vi "All on BAP4B.vi"(8 "mode set":T3, 10 "system state in":T1) -> (2 "system state out":T1)   [LabVIEW 2014]
doc: "All on BAP4B\n\nSets all the lights on for the All On Test according to the mode. Updates the system state.\n\nBeverly Abadines\nPHY 350\nP4"
uses:
  typedefs/control mode enum.ctl
  typedefs/system state cluster.ctl
  typedefs/state enum.ctl
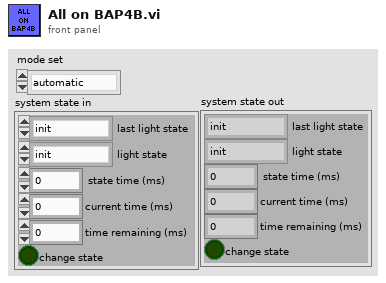
[diagram p1: front panel]
types:
  T1 = typedef "system state cluster.ctl" = cluster{"last light state":T2, "light state":T2, "state time (ms)":i32, "current time (ms)":i32, "time remaining (ms)":i32, "change state":bool}
  T2 = typedef "state enum.ctl" = enum16{"init", "idle", "left turn E", "go EW", "caution EW", "left turn W", "left turn N", "go NS", "caution NS", "left turn S", "blink on", "blink off", "all on test", "exit"}
  T3 = typedef "control mode enum.ctl" = enum16{"automatic", "blinking", "all on test"}
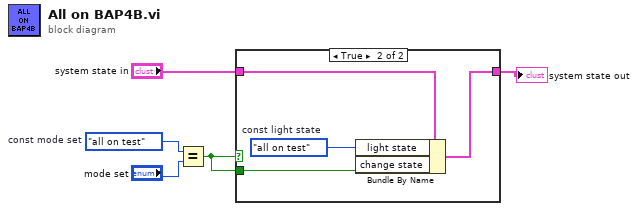
[diagram p0: block diagram]
diagram:
  w3 = control_mode_enum."all on test"  # const mode set
  n1 = Equal?(x=w3, y="mode set") -> (x = y?=w2:bool)
  n2 = case shown="True" w2 {
    tunnel: "system state in" -> [w6 w10]
    tunnel: w2 -> [_ w9]
    tunnel: [w6 w8] -> w1
    frame False {
    }
    frame True {
      w7 = state_enum."all on test"  # const light state
      n3 = Bundle By Name(cluster=w10, "light state"=w7, "change state"=w9) -> (w8:T1)
    }
  }
  "system state out" <- w1
